vi "Get_19572_total_test_time.vi"(8 "error in (no error)":errorcluster, 11 "VISA resource in":refnum<visa-resource-name>) -> (0 "error out":errorcluster, 2 "Data":T1, 3 "VISA resource out":refnum<visa-resource-name>)   [LabVIEW 2015]
doc: "This VI calculates the test time of the 19052 Hi-Pot instrument, considering that the test step(s) may consist of (some or all) AC, DC and IR tests, regardless of the number of steps, repetition or order of occurrence."
uses:
  Type Definitions/get_19572_total_test_time_states.ctl
panel:
  # "19572 Ground Bond Tester\nGet Total Test Time"
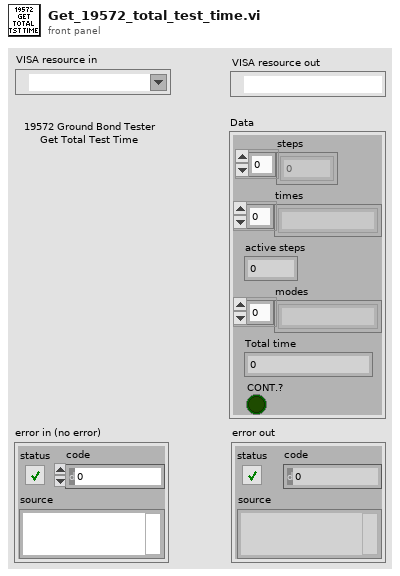
[diagram p1: front panel]
types:
  T1 = cluster{"steps":u16[], "times":string[], "active steps":u16, "modes":string[], "Total time":dbl, "CONT.?":bool}
  T2 = typedef "get_19572_total_test_time_states.ctl" = enum16{"Initialize", "get active STEPs", "get active MODEs", "Get STEPs time", "check CONT.", "get TOTAL time", "Error", "Shutdown"}
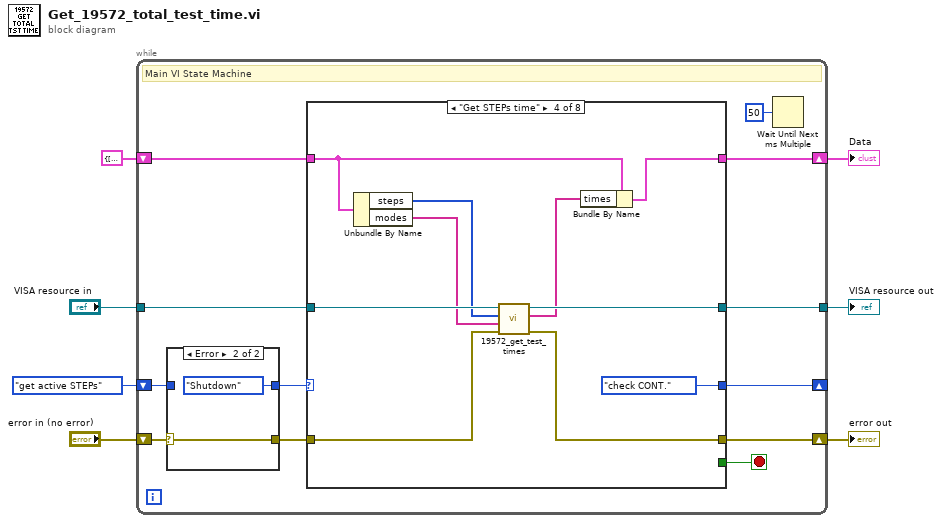
[diagram p0: block diagram]
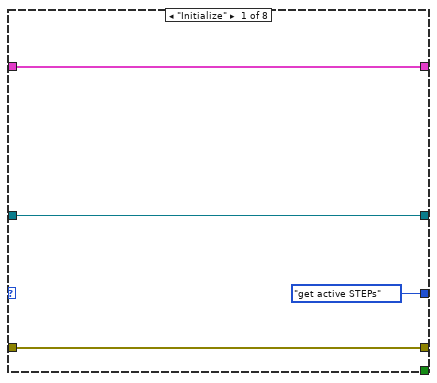
[diagram p3: hidden frame]
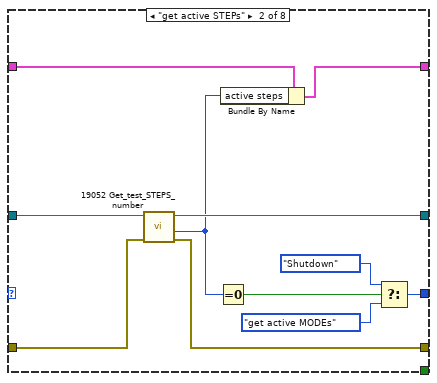
[diagram p4: hidden frame]
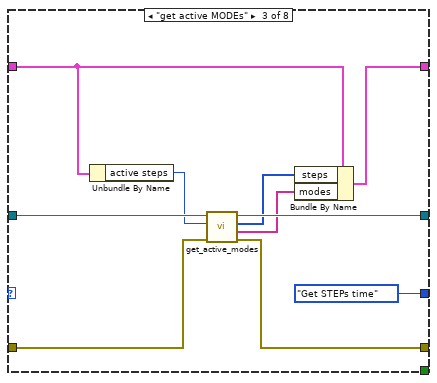
[diagram p5: hidden frame]
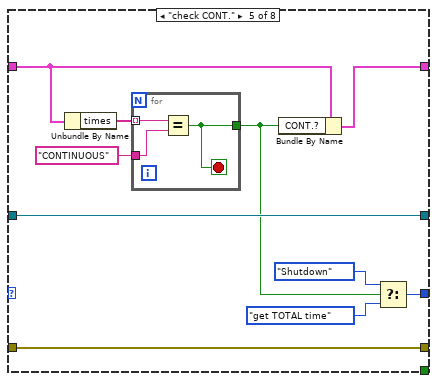
[diagram p6: hidden frame]
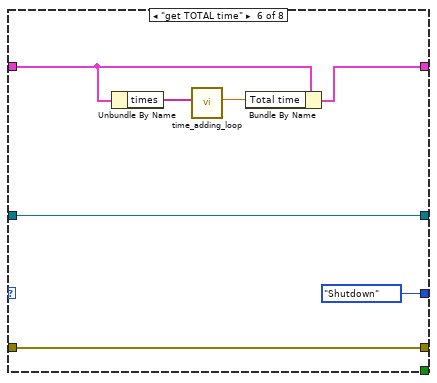
[diagram p7: hidden frame]
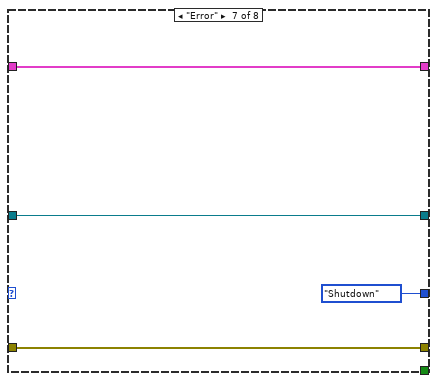
[diagram p8: hidden frame]
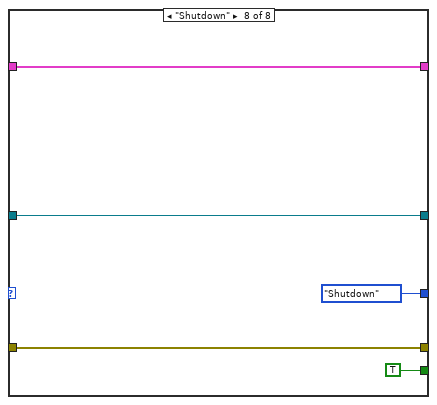
[diagram p9: hidden frame]
diagram:
  n1 = while {
    shift-right: [w19] -> _
    shift-left: get_19572_total_test_time_states."get active STEPs" -> [w9]
    tunnel: "VISA resource in" -> [w18]
    tunnel: [w17] -> w2
    shift-right: [w16] -> w1
    shift-left: "error in (no error)" -> [w12]
    shift-right: [w13] -> w4
    shift-left: T1 {"steps"=[], "times"=[], "active steps"=0, "modes"=[], "Total time"=0.0, "CONT.?"=FALSE} -> [w14]
    stop <- w15 stop-if-true
    # "Main VI State Machine"
    n2 = case shown="Error" w12 {
      selector: w12 -> [w21 w23]
      tunnel: [w21 w23] -> w11
      tunnel: [w20 get_19572_total_test_time_states."Shutdown"] -> w10
      tunnel: w9 -> [w20 _]
      frame No Error {
      }
      frame Error {
      }
    }
    n3 = case shown="\"Get STEPs time\"" w10 {
      tunnel: [get_19572_total_test_time_states."get active STEPs" w33 get_19572_total_test_time_states."Get STEPs time" get_19572_total_test_time_states."check CONT." w65 get_19572_total_test_time_states."Shutdown" get_19572_total_test_time_states."Shutdown" get_19572_total_test_time_states."Shutdown"] -> w19
      tunnel: w18 -> [w26 w37 w47 w56 w68 w74 w82 w84]
      tunnel: [w26 w38 w48 w53 w68 w74 w82 w84] -> w17
      tunnel: w11 -> [w25 w36 w46 w55 w67 w78 w81 w86]
      tunnel: [w25 w35 w42 w54 w67 w78 w81 w86] -> w16
      tunnel: [_ _ _ _ _ _ _ TRUE] -> w15
      tunnel: w14 -> [w27 w30 w40 w51 w61 w76 w80 w87]
      tunnel: [w27 w28 w45 w57 w60 w75 w80 w87] -> w13
      frame "Initialize" {
      }
      frame "get active STEPs" {
        n4 = call "19052 Get_test_STEPS_number.vi"("error in (no error)"=w36, "VISA resource in"=w37) -> ("error out"=w35:errorcluster, "# Active steps"=w29:u16, "VISA resource out"=w38:refnum<visa-resource-name>)  [unwired: 7 in]
        n5 = Equal To 0?(x=w29) -> (x = 0?=w34:bool)
        n6 = Bundle By Name(cluster=w30, "active steps"=w29) -> (w28:T1)
        n7 = Select(t=get_19572_total_test_time_states."Shutdown", s=w34, f=get_19572_total_test_time_states."get active MODEs") -> (s? t:f=w33:T2)
      }
      frame "get active MODEs" {
        n8 = Unbundle By Name(w40) -> ("active steps"=w39:u16)
        n9 = call "get_active_modes.vi"("error in (no error)"=w46, "active steps"=w39, "VISA Refnum in"=w47) -> ("error out"=w42:errorcluster, "modes"=w43:string[], "steps"=w44:u16[], "VISA Refnum out"=w48:refnum<visa-resource-name>)  [unwired: 5 in]
        n10 = Bundle By Name(cluster=w40, "steps"=w44, "modes"=w43) -> (w45:T1)
      }
      frame "Get STEPs time" {
        n11 = Unbundle By Name(w51) -> ("steps"=w49:u16[], "modes"=w50:string[])
        n12 = call "19572_get_test_times.vi"("error in (no error)"=w55, "modes"=w50, "steps"=w49, "VISA Refnum in"=w56) -> ("error out"=w54:errorcluster, "times"=w52:string[], "VISA Refnum out"=w53:refnum<visa-resource-name>)  [unwired: 5 in]
        n13 = Bundle By Name(cluster=w51, "times"=w52) -> (w57:T1)
      }
      frame "check CONT." {
        n14 = Unbundle By Name(w61) -> ("times"=w66:string[])
        n15 = for {
          tunnel: w66 -> [w71] mode=indexing
          tunnel: [w70] -> w59
          tunnel: "CONTINUOUS" -> [w69]
          stop <- w70 stop-if-true
          n16 = Equal?(x=w71, y=w69) -> (x = y?=w70:bool)
        }
        n17 = Bundle By Name(cluster=w61, "CONT.?"=w59) -> (w60:T1)
        n18 = Select(t=get_19572_total_test_time_states."Shutdown", s=w59, f=get_19572_total_test_time_states."get TOTAL time") -> (s? t:f=w65:T2)
      }
      frame "get TOTAL time" {
        n19 = Unbundle By Name(w76) -> ("times"=w73:string[])
        n20 = call "time_adding_loop.vi"("times"=w73) -> ("Total time"=w72:dbl)  [unwired: 10 in]
        n21 = Bundle By Name(cluster=w76, "Total time"=w72) -> (w75:T1)
      }
      frame "Error" {
      }
      frame "Shutdown" {
      }
    }
    n22 = Wait Until Next ms Multiple(millisecond multiple=u32 50) -> ()  [unwired: 1 out]
  }
  "error out" <- w1
  "VISA resource out" <- w2
  "Data" <- w4
